vi "Init log file.vi"(8 "error in (no error)":errorcluster, 11 "Channel in":refnum<class "SPARC4_Channel.lvclass">) -> (0 "error out":errorcluster, 3 "Channel out":refnum<class "SPARC4_Channel.lvclass">)   [LabVIEW 2018, in "SPARC4_Channel.lvclass"]
uses:
  SPARC4_Channel.lvclass
  Log File/Log File.lvclass
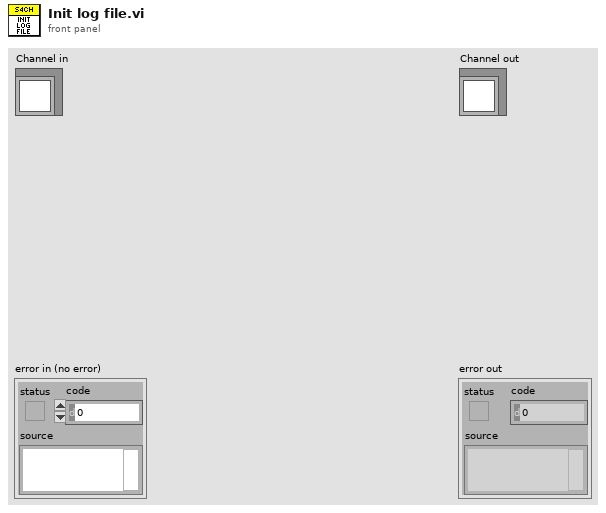
[diagram p1: front panel]
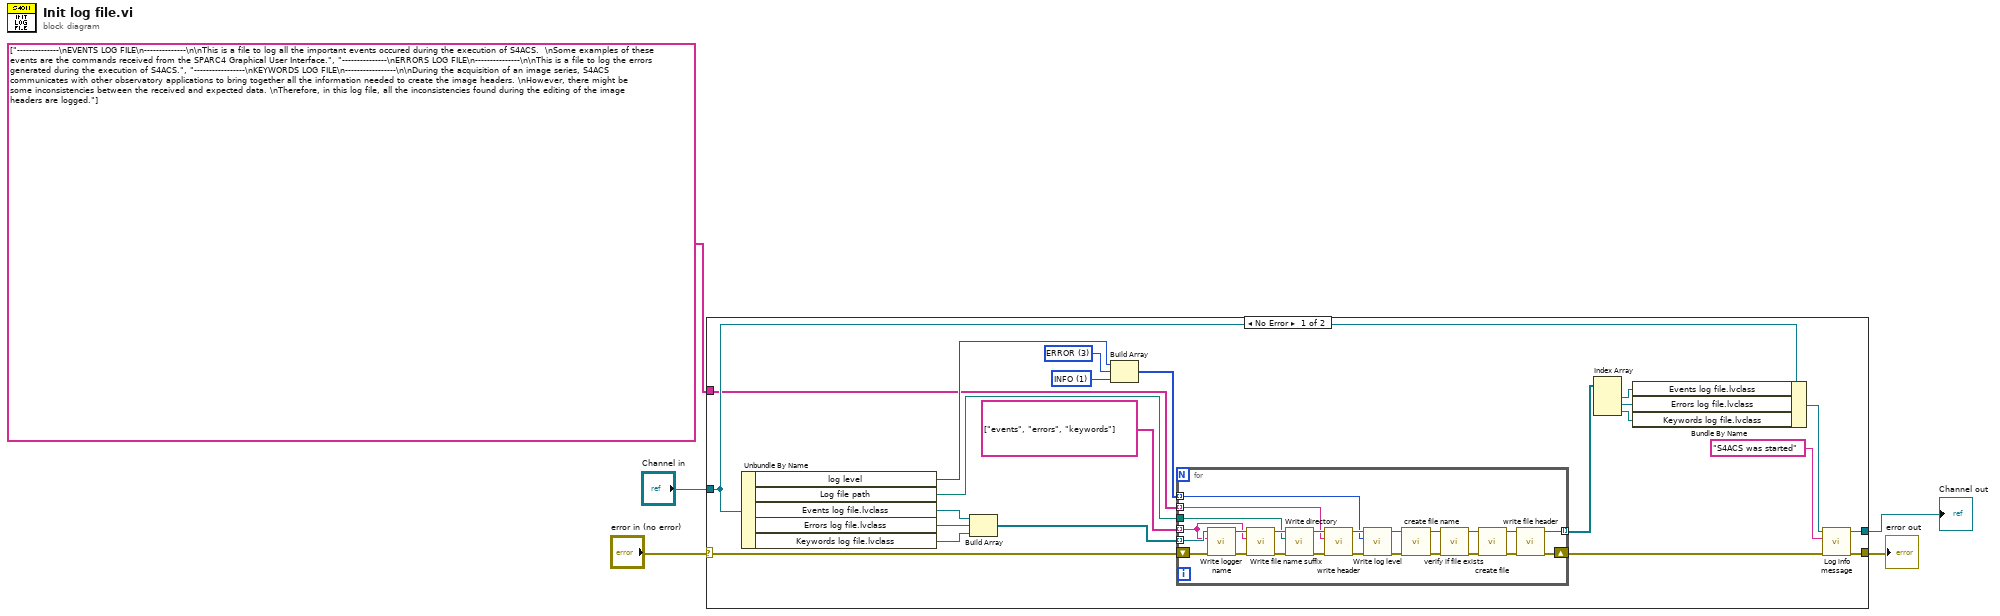
[diagram p0: block diagram]
diagram:
  n1 = case shown="No Error" "error in (no error)" {
    selector: "error in (no error)" -> [w27 w53]
    tunnel: [w8 w53] -> w4
    tunnel: [w9 w52] -> w2
    tunnel: "Channel in" -> [w26 w52]
    tunnel: string[] ["--------------\nEVENTS LOG FILE\n--------------\n\nThis is a file to log all the important events occured during the execution of S4ACS.  \nSome examples of these events are the commands received from the SPARC4 Graphical User Interface.", "---------------\nERRORS LOG FILE\n---------------\n\nThis is a file to log the errors generated during the execution of S4ACS.", "-----------------\nKEYWORDS LOG FILE\n-----------------\n\nDuring the acquisition of an image series, S4ACS communicates with other observatory applications to bring together all the information needed to create the image headers. \nHowever, there might be some inconsistencies between the received and expected data. \nTherefore, in this log file, all the inconsistencies found during the editing of the image headers are logged."] -> [w12 _]
    frame No Error {
      w16 = u16 1 items=["DEBBUG", "INFO", "WARNING", "ERROR", "CRITICAL"] ("log level")
      w17 = u16 3 items=["DEBBUG", "INFO", "WARNING", "ERROR", "CRITICAL"] ("log level")
      n2 = Unbundle By Name(w26) -> ("log level"=w15:u16, "Log file path"=w13:path, "Events log file.lvclass"=w25:refnum<class "Log File.lvclass">, "Errors log file.lvclass"=w24:refnum<class "Log File.lvclass">, "Keywords log file.lvclass"=w23:refnum<class "Log File.lvclass">)
      n3 = Build Array(w25, w24, w23) -> (w22:refnum<class "Log File.lvclass">[])
      n4 = Build Array(w15, w17, w16) -> (w14:u16[])
      n5 = for {
        shift-right: [w37] -> w7
        shift-left: w27 -> [w33]
        tunnel: w22 -> [w36] mode=indexing
        tunnel: string[] ["events", "errors", "keywords"] -> [w32] mode=indexing
        tunnel: [w31] -> w20 mode=indexing
        tunnel: w14 -> [w30] mode=indexing
        tunnel: w13 -> [w29]
        tunnel: w12 -> [w28] mode=indexing
        n6 = call-dynamic "Write logger name.vi"("error in (no error)"=w33, "logger name"=w32, "Log File in"=w36) -> ("error out"=w34:errorcluster, "Log File out"=w35:refnum<class "Log File.lvclass">)  [unwired: 7 in]
        n7 = call-dynamic "Write file name suffix.vi"("error in (no error)"=w34, "file name suffix"=w32, "Log File in"=w35) -> ("error out"=w46:errorcluster, "Log File out"=w47:refnum<class "Log File.lvclass">)  [unwired: 7 in]
        n8 = call "Write directory.vi"("error in (no error)"=w46, "log dir"=w29, "Log File in"=w47) -> ("error out"=w50:errorcluster, "Log File out"=w51:refnum<class "Log File.lvclass">)  [unwired: 7 in]
        n9 = call "write header.vi"("error in (no error)"=w50, "header"=w28, "Log File in"=w51) -> ("error out"=w38:errorcluster, "Log File out"=w41:refnum<class "Log File.lvclass">)  [unwired: 7 in]
        n10 = call-dynamic "Write log level.vi"("error in (no error)"=w38, "log level"=w30, "Log File in"=w41) -> ("error out"=w39:errorcluster, "Log File out"=w40:refnum<class "Log File.lvclass">)  [unwired: 7 in]
        n11 = call "create file name.vi"("error in (no error)"=w39, "Log File in"=w40) -> ("error out"=w45:errorcluster, "Log File out"=w44:refnum<class "Log File.lvclass">)  [unwired: 8 in]
        n12 = call-dynamic "verify if file exists.vi"("error in (no error)"=w45, "Log File in"=w44) -> ("error out"=w42:errorcluster, "Log File out"=w43:refnum<class "Log File.lvclass">)  [unwired: 8 in]
        n13 = call "create file.vi"("error in (no error)"=w42, "Log File in"=w43) -> ("error out"=w48:errorcluster, "Log File out"=w49:refnum<class "Log File.lvclass">)  [unwired: 8 in]
        n14 = call-dynamic "write file header.vi"("error in (no error)"=w48, "Log File in"=w49) -> ("error out"=w37:errorcluster, "Log File out"=w31:refnum<class "Log File.lvclass">)  [unwired: 8 in]
      }
      n15 = Index Array(array=w20) -> (element #1=w11:refnum<class "Log File.lvclass">, element #2=w19:refnum<class "Log File.lvclass">, element #3=w18:refnum<class "Log File.lvclass">)  [unwired: 3 in]
      n16 = Bundle By Name(cluster=w26, "Events log file.lvclass"=w11, "Errors log file.lvclass"=w19, "Keywords log file.lvclass"=w18) -> (w10:refnum<class "SPARC4_Channel.lvclass">)
      n17 = call "Log info message.vi"("error in (no error)"=w7, "String"="S4ACS was started" ("Message to log"), "Channel in"=w10) -> ("error out"=w8:errorcluster, "Channel out"=w9:refnum<class "SPARC4_Channel.lvclass">)  [unwired: 7 in]
    }
    frame Error {
    }
  }
  "error out" <- w4
  "Channel out" <- w2
